vi "unmarshalling.vi"(7 "Type":variant, 8 "error in (no error)":errorcluster, 10 "String":string, 11 "Serializer":refnum<class "Serializer.PlainText.lvclass">) -> (0 "error out":errorcluster, 2 "Variant":variant, 3 "Serializer out":refnum<class "Serializer.PlainText.lvclass">)   [LabVIEW 2013, in "Serializer.PlainText.lvclass"]
uses:
  Serializer.PlainText.lvclass
  <vilib>/LabVIEW Open Source Project/Data Manipulation/TypeDescriptor/TypeDescriptor_GetName.vi
  <vilib>/LabVIEW Open Source Project/Data Manipulation/TypeDescriptor/TypeDescriptor_GetType.vi
  <vilib>/LabVIEW Open Source Project/Data Manipulation/TypeDescriptor/TypeDescriptor_GetPString.vi
  <vilib>/Utility/GetType.llb/TD_Create Cluster.vi
  <vilib>/Utility/GetType.llb/TD_Get Array Information.vi
  <vilib>/Utility/GetType.llb/Get Type Code from I16 Array And Pos.vi
  <vilib>/LabVIEW Open Source Project/Data Manipulation/TypeDescriptor/TypeDescriptor_SetName.vi
  <vilib>/LabVIEW Open Source Project/Data Manipulation/Variant/OpenVariant.lvlib
  <vilib>/Utility/VariantDataType/VariantType.lvlib
  <vilib>/LabVIEW Open Source Project/Data Manipulation/TypeDescriptor/OpenDescriptor.lvlib
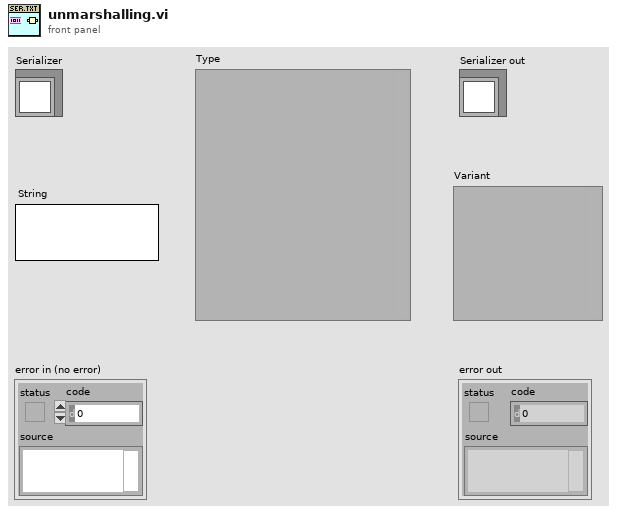
[diagram p1: front panel]
types:
  T1 = typedef "VariantType.lvlib/Type.ctl" = enum8{"Invalid Type", "Void", "I8", "I16", "I32", "I64", "U8", "U16", "U32", "U64", "Single Float", "Double Float", "Extended Float", "Single Complex", "Double Complex", "Extended Complex", "Enum U8", "Enum U16", "Enum U32", "Enum U64", "Single Float With Unit", "Double Float With Unit", "Extended Float With Unit", "Single Complex with Unit", "Double Complex with Unit", "Extended Complex with Unit", "Boolean", "String", "Path", "Picture", "Tag", "Array", "Cluster", "Variant", "LV Variant", "Waveform", "Timestamp", "Digital Waveform", "Digital Data", "ExpressData", "Refnum", "External Data", "VI", "Poly VI", "LabVIEW Class Instance", "Fixed Point"}
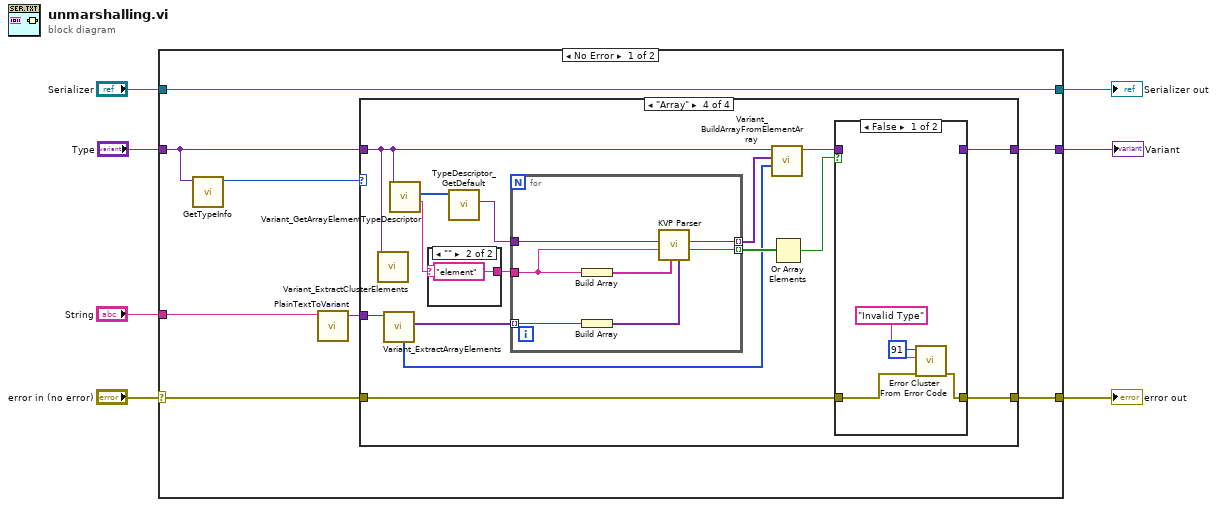
[diagram p0: block diagram]
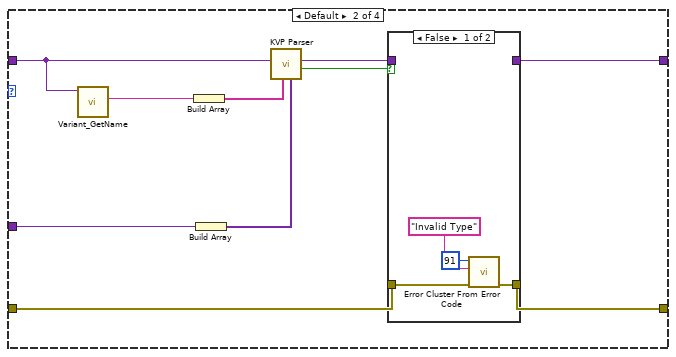
[diagram p3: hidden frame]
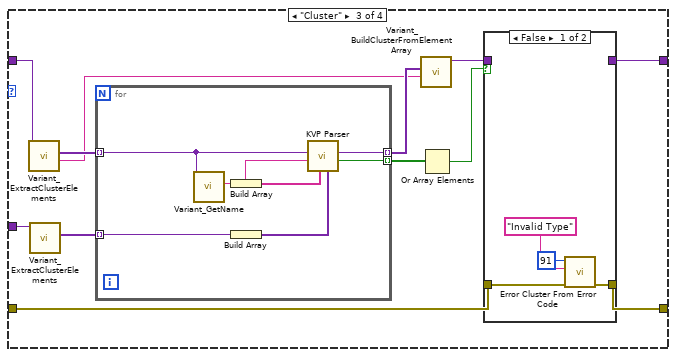
[diagram p5: hidden frame]
diagram:
  n1 = case shown="No Error" "error in (no error)" {
    selector: "error in (no error)" -> [w12 w90]
    tunnel: [w11 w90] -> w6
    tunnel: [w10 w89] -> w4
    tunnel: "Serializer" -> [w10 w89]
    tunnel: [w14 _] -> w3
    tunnel: "Type" -> [w13 _]
    tunnel: "String" -> [w9 _]
    frame No Error {
      n2 = call <vilib>:"GetTypeInfo.vi"("Variant"=w13) -> ("Type Enum"=w8:T1)  [unwired: 6 in, 4 out]
      n3 = call "PlainTextToVariant.vi"("String-formatted Value"=w9) -> ("Variant-formatted Value"=w15:variant)  [unwired: 9 in, 1 out]
      n4 = case shown="\"Array\"" w8 {
        tunnel: w15 -> [w17 w25 w42 w67]
        tunnel: [w17 w20 w45 w73] -> w14
        tunnel: w13 -> [_ w23 w41 w61]
        tunnel: w12 -> [w16 w18 w43 w71]
        tunnel: [w16 w19 w44 w72] -> w11
        frame "Void" {
        }
        frame Default {
          n5 = call <vilib>:"Variant_GetName.vi"("Variant"=w23) -> ("Name"=w27:string)  [unwired: 8 in, 2 out]
          n6 = Build Array(w27) -> (w26:string[])
          n7 = Build Array(w25) -> (w24:variant[])
          n8 = call <vilib>:"KVP Parser.vi"("Values"=w24, "Keys"=w26, "Default Value"=w23) -> ("any found?"=w22:bool, "Value"=w21:variant)  [unwired: 5 in, 2 out]
          n9 = case shown="False" w22 {
            tunnel: w21 -> [_ w33]
            tunnel: [_ w33] -> w20
            tunnel: [w31 w32] -> w19
            tunnel: w18 -> [w30 w32]
            frame False {
              n10 = call <vilib>:"Error Cluster From Error Code.vi"("error in (no error)"=w30, "error message (\"\")"="Invalid Type", "error code (0)"=91) -> ("error out"=w31:errorcluster)  [unwired: 6 in]
            }
            frame True {
            }
          }
        }
        frame "Cluster" {
          n11 = call <vilib>:"Variant_ExtractClusterElements.vi"("Cluster"=w41) -> ("name"=w37:string, "Elements"=w40:variant[])  [unwired: 8 in, 1 out]
          n12 = call <vilib>:"Variant_ExtractClusterElements.vi"("Cluster"=w42) -> ("Elements"=w39:variant[])  [unwired: 8 in, 2 out]
          n13 = for {
            tunnel: w40 -> [w52] mode=indexing
            tunnel: w39 -> [w49] mode=indexing
            tunnel: [w51] -> w38 mode=indexing
            tunnel: [w50] -> w35 mode=indexing
            n14 = call <vilib>:"Variant_GetName.vi"("Variant"=w52) -> ("Name"=w46:string)  [unwired: 8 in, 2 out]
            n15 = Build Array(w46) -> (w48:string[])
            n16 = Build Array(w49) -> (w47:variant[])
            n17 = call <vilib>:"KVP Parser.vi"("Values"=w47, "Keys"=w48, "Default Value Name (empty: label)"=w46, "Default Value"=w52) -> ("any found?"=w50:bool, "Value"=w51:variant)  [unwired: 4 in, 2 out]
          }
          n18 = call <vilib>:"Variant_BuildClusterFromElementArray.vi"("name"=w37, "Elements"=w38) -> ("Cluster"=w36:variant)  [unwired: 9 in]
          n19 = Or Array Elements(Boolean array=w35) -> (logical OR=w34:bool)
          n20 = case shown="False" w34 {
            tunnel: w36 -> [_ w58]
            tunnel: [_ w58] -> w45
            tunnel: [w56 w57] -> w44
            tunnel: w43 -> [w55 w57]
            frame False {
              n21 = call <vilib>:"Error Cluster From Error Code.vi"("error in (no error)"=w55, "error message (\"\")"="Invalid Type", "error code (0)"=91) -> ("error out"=w56:errorcluster)  [unwired: 6 in]
            }
            frame True {
            }
          }
        }
        frame "Array" {
          n22 = call <vilib>:"Variant_ExtractClusterElements.vi"("Cluster"=w61) -> ()  [unwired: 8 in, 3 out]
          n23 = call <vilib>:"Variant_ExtractArrayElements.vi"("Array"=w67) -> ("Elements"=w66:variant[], "Dimensions"=w62:u32[])  [unwired: 7 in, 2 out]
          n24 = call <vilib>:"Variant_GetArrayElementTypeDescriptor.vi"("Array"=w61) -> ("Element Name"=w60:string, "Element Descriptor"=w68:i16[])  [unwired: 8 in, 1 out]
          n25 = case shown="\"\"" w60 {
            selector: w60 -> [w74 _]
            tunnel: [w74 "element"] -> w59
            frame Default {
            }
            frame "" {
            }
          }
          n26 = call <vilib>:"TypeDescriptor_GetDefault.vi"("type descriptor"=w68) -> ("Default"=w65:variant)  [unwired: 8 in, 2 out]
          n27 = for {
            tunnel: w65 -> [w82]
            tunnel: w66 -> [w79] mode=indexing
            tunnel: [w81] -> w63 mode=indexing
            tunnel: [w80] -> w70 mode=indexing
            tunnel: w59 -> [w76]
            n28 = Build Array(w76) -> (w78:string[])
            n29 = Build Array(w79) -> (w77:variant[])
            n30 = call <vilib>:"KVP Parser.vi"("Values"=w77, "Keys"=w78, "Default Value Name (empty: label)"=w76, "Default Value"=w82) -> ("any found?"=w80:bool, "Value"=w81:variant)  [unwired: 4 in, 2 out]
          }
          n31 = call <vilib>:"Variant_BuildArrayFromElementArray.vi"("Dimensions"=w62, "Elements"=w63, "Default Array"=w61) -> ("Output Array"=w64:variant)  [unwired: 7 in, 1 out]
          n32 = Or Array Elements(Boolean array=w70) -> (logical OR=w69:bool)
          n33 = case shown="False" w69 {
            tunnel: w64 -> [_ w88]
            tunnel: [_ w88] -> w73
            tunnel: [w86 w87] -> w72
            tunnel: w71 -> [w85 w87]
            frame False {
              n34 = call <vilib>:"Error Cluster From Error Code.vi"("error in (no error)"=w85, "error message (\"\")"="Invalid Type", "error code (0)"=91) -> ("error out"=w86:errorcluster)  [unwired: 6 in]
            }
            frame True {
            }
          }
        }
      }
    }
    frame Error {
    }
  }
  "error out" <- w6
  "Serializer out" <- w4
  "Variant" <- w3
